vi "Send 485 Command.vi"(6 "CIB address":string="1", 10 "COM Ref":refnum<visa-resource-name>, 11 "Message":string="help") -> (0 "Error Out":errorcluster)   [LabVIEW 2013]
uses:
  RS485/Port Config.ctl
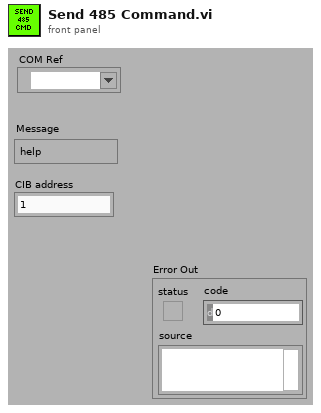
[diagram p1: front panel]
types:
  T1 = typedef "Port Config.ctl" = cluster{"VISA resource name":refnum<visa-resource-name>, "baud rate":u32, "data bits (8)":u16, "parity (0:none)":enum16{"None", "Odd", "Even", "Mark", "Space"}, "stop bits (10: 1 bit)":u16, "flow control (0:none)":u16, "timeout (2sec)":u32}
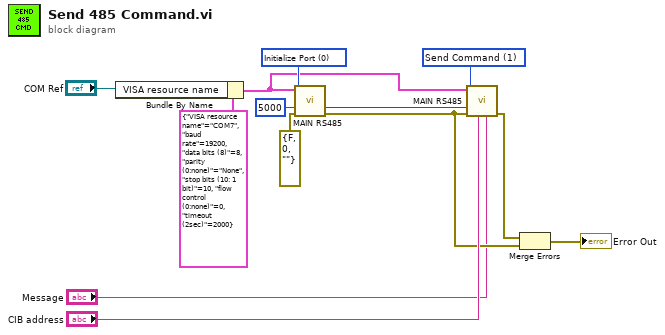
[diagram p0: block diagram]
diagram:
  w8 = u16 1 items=["Initialize Port", "Send Command", "Get Commands"] ("RS485 Operation")
  w2 = u32 5000 ("Timeout (ms)")
  w9 = u16 0 items=["Initialize Port", "Send Command", "Get Commands"] ("RS485 Operation")
  n1 = Bundle By Name(cluster=T1 {"VISA resource name"="COM7", "baud rate"=19200, "data bits (8)"=8, "parity (0:none)"=enum."None", "stop bits (10: 1 bit)"=10, "flow control (0:none)"=0, "timeout (2sec)"=2000} ("PortConfig"), "VISA resource name"="COM Ref") -> (w3:T1)
  n2 = call "MAIN RS485.vi"("Error In"=errorcluster {"status"=FALSE, "code"=0, "source"=""}, "Timeout (ms)"=w2, "RS485 Operation"=w9, "PortConfig"=w3) -> ("Error Out"=w5:errorcluster)  [unwired: 6 in, 1 out]
  n3 = call "MAIN RS485.vi"("message"="Message", "CIB address"="CIB address", "Error In"=w5, "Timeout (ms)"=w2, "RS485 Operation"=w8, "PortConfig"=w3) -> ("Error Out"=w6:errorcluster)  [unwired: 4 in, 1 out]
  n4 = Merge Errors(w6, w5) -> (→"Error Out":errorcluster)
